vi "parseDataDBL.vi"(8 "error in (no error)":errorcluster, 11 "FrameParser in":refnum<class "FrameParser.lvclass">) -> (0 "error out":errorcluster, 2 "Data":dbl, 3 "FrameParser out":refnum<class "FrameParser.lvclass">)   [LabVIEW 2015, in "FrameParser.lvclass"]
uses:
  FrameParser.lvclass
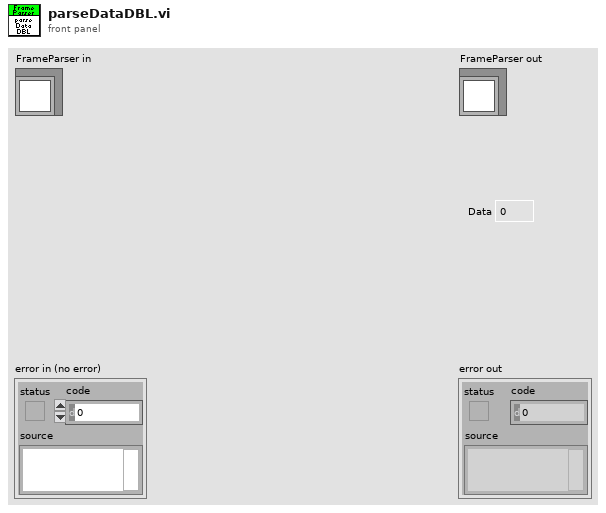
[diagram p1: front panel]
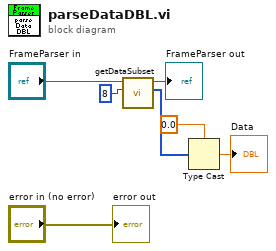
[diagram p0: block diagram]
diagram:
  n1 = call "getDataSubset.vi"("Length"=8 ("Count"), "FrameParser in"="FrameParser in") -> ("Data"=w2:u8[], "FrameParser out"=→"FrameParser out":refnum<class "FrameParser.lvclass">)  [unwired: 7 in, 1 out]
  n2 = Type Cast(type=0.0, x=w2) -> (*(type *) &x=→"Data":dbl)
  "error out" <- "error in (no error)"
